vi "Vib Readout.vi"(8 "error in":errorcluster, 11 "DAC HS Vib in":refnum<class "DAC HS Vib.lvclass">) -> (0 "error out":errorcluster, 3 "DAC HS Vib out":refnum<class "DAC HS Vib.lvclass">)   [LabVIEW 2019, in "DAC.lvlib" / "DAC HS Vib.lvclass"]
uses:
  DAC HS Vib.lvclass
  DAC.lvclass
  <vilib>/DAQmx/read.llb/DAQmx Read (Analog DBL 1Chan 1Samp).vi
  <vilib>/DAQmx/read.llb/DAQmx Read (Analog Wfm 1Chan NSamp).vi
  Results/Results Method.ctl
  Results/Results.lvlib
  Results/DeepU Results/DeepU Results.lvclass
  C:/Users/krio/Documents/LV_Projects/test-stand/App/DAC/DAC.lvclass
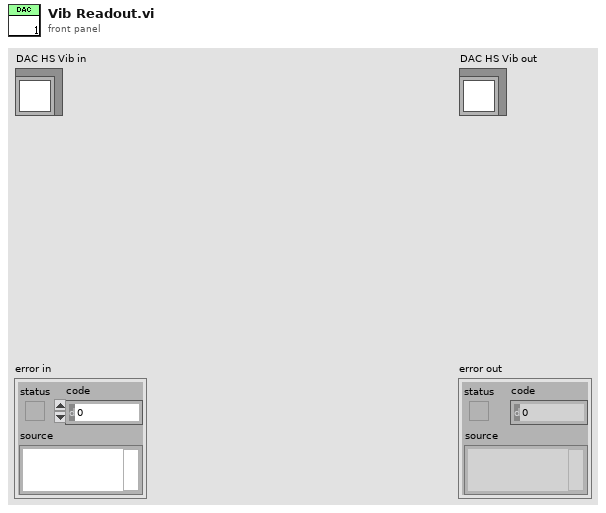
[diagram p1: front panel]
types:
  T1 = typedef "Results.lvlib/Results Method.ctl" = enum16{"Get", "Set"}
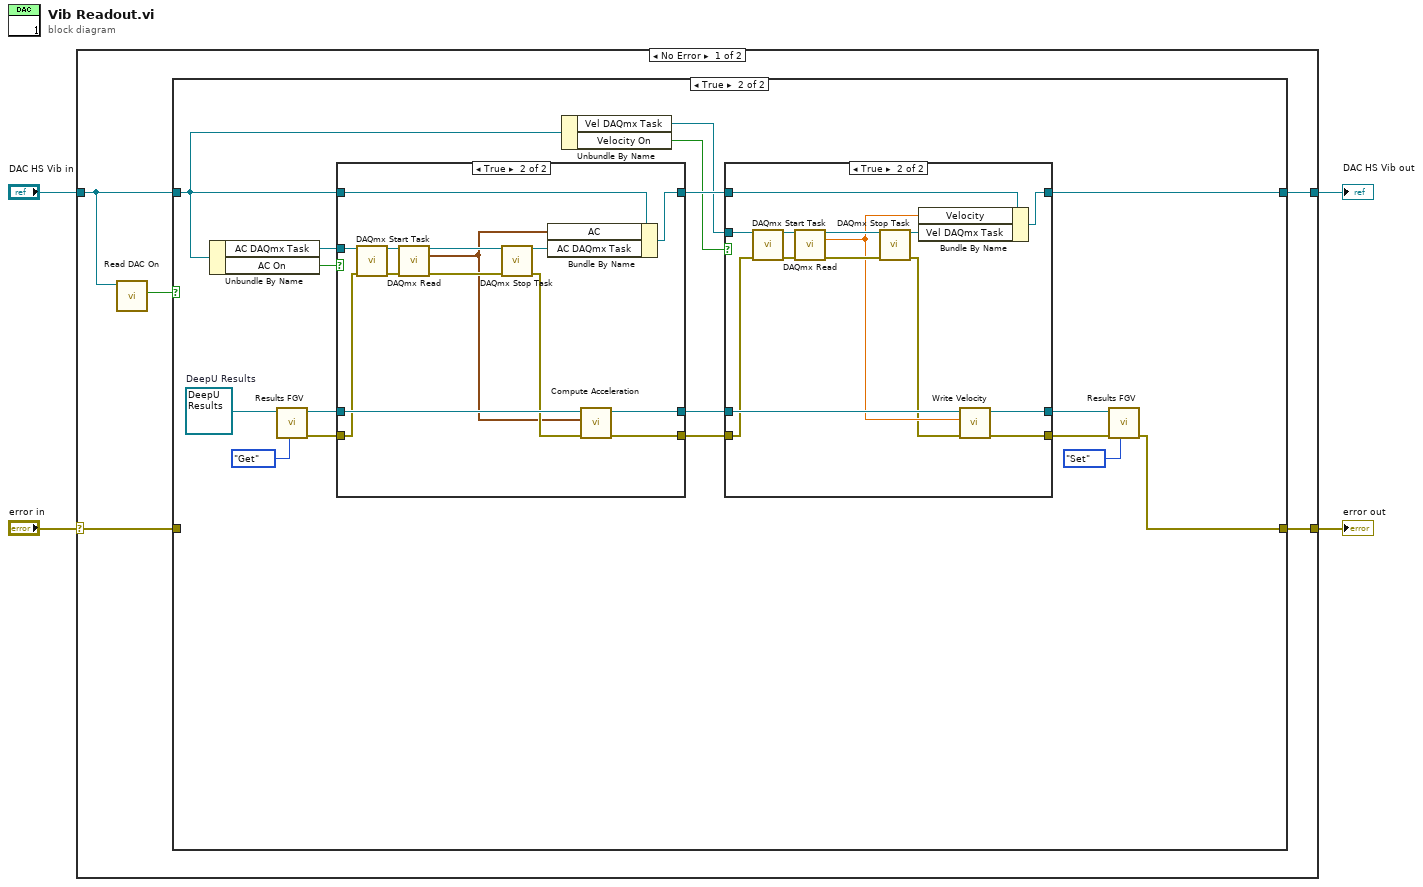
[diagram p0: block diagram]
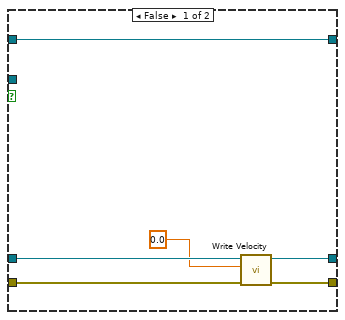
[diagram p3: hidden frame]
diagram:
  n1 = case shown="No Error" "error in" {
    selector: "error in" -> [w5 w67]
    tunnel: [w6 w67] -> w3
    tunnel: [w7 w66] -> w1
    tunnel: "DAC HS Vib in" -> [w8 w66]
    frame No Error {
      n2 = call "Read DAC On.vi"("DAC in"=w8) -> ("DAC On"=w9:bool)  [unwired: 8 in, 2 out]
      n3 = case shown="True" w9 {
        tunnel: w8 -> [w11 w25]
        tunnel: [w11 w27] -> w7
        tunnel: w5 -> [w10 _]
        tunnel: [w10 w15] -> w6
        frame False {
        }
        frame True {
          w21 = refnum<class "DeepU Results.lvclass"> refnum  # DeepU Results
          n4 = Unbundle By Name(w25) -> ("AC DAQmx Task"=w26:refnum<k21>, "AC On"=w24:bool)
          n5 = call-dynamic "Results FGV.vi"("Method"=Results_Method."Get", "DeepU Results in"=w21) -> ("error out"=w12:errorcluster, "DeepU Results out"=w18:refnum<class "DeepU Results.lvclass">)  [unwired: 8 in]
          n6 = case shown="True" w24 {
            tunnel: w25 -> [w51 w65]
            tunnel: [w51 w64] -> w28
            tunnel: w26 -> [_ w63]
            tunnel: w18 -> [w50 w57]
            tunnel: [w50 w56] -> w17
            tunnel: [w49 w54] -> w13
            tunnel: w12 -> [w49 w53]
            frame False {
            }
            frame True {
              n7 = call <vilib>:"DAQmx Start Task.vi"("task/channels in"=w63, "error in"=w53) -> ("task out"=w62:refnum<k21>, "error out"=w59:errorcluster)  [unwired: 12 in]
              n8 = call-poly <vilib>:"DAQmx Read.vi"("task/channels in"=w62, "error in"=w59) -> ("task out"=w61:refnum<k21>, "data"=w52:waveform(dbl), "error out"=w58:errorcluster)  [unwired: 11 in]
              n9 = call <vilib>:"DAQmx Stop Task.vi"("task/channels in"=w61, "error in"=w58) -> ("task out"=w60:refnum<k21>, "error out"=w55:errorcluster)  [unwired: 12 in]
              n10 = Bundle By Name(cluster=w65, "AC"=w52, "AC DAQmx Task"=w60) -> (w64:refnum<class "DAC HS Vib.lvclass">)
              n11 = call "Compute Acceleration.vi"("error in"=w55, "AC"=w52, "DeepU Results in"=w57) -> ("error out"=w54:errorcluster, "DeepU Results out"=w56:refnum<class "DeepU Results.lvclass">)  [unwired: 7 in]
            }
          }
          n12 = Unbundle By Name(w25) -> ("Vel DAQmx Task"=w22:refnum<k21>, "Velocity On"=w23:bool)
          n13 = case shown="True" w23 {
            tunnel: [w34 w48] -> w27
            tunnel: w28 -> [w34 w47]
            tunnel: w22 -> [_ w46]
            tunnel: w17 -> [w33 w40]
            tunnel: [w32 w38] -> w16
            tunnel: [w29 w36] -> w14
            tunnel: w13 -> [w30 w35]
            frame False {
              n14 = call "Write Velocity.vi"("error in (no error)"=w30, "Velocity"=0.0, "DeepU Results in"=w33) -> ("error out"=w29:errorcluster, "DeepU Results out"=w32:refnum<class "DeepU Results.lvclass">)  [unwired: 7 in]
            }
            frame True {
              n15 = call <vilib>:"DAQmx Start Task.vi"("task/channels in"=w46, "error in"=w35) -> ("task out"=w45:refnum<k21>, "error out"=w42:errorcluster)  [unwired: 12 in]
              n16 = call-poly <vilib>:"DAQmx Read.vi"("task/channels in"=w45, "error in"=w42) -> ("task out"=w44:refnum<k21>, "data"=w39:dbl, "error out"=w41:errorcluster)  [unwired: 11 in]
              n17 = call <vilib>:"DAQmx Stop Task.vi"("task/channels in"=w44, "error in"=w41) -> ("task out"=w43:refnum<k21>, "error out"=w37:errorcluster)  [unwired: 12 in]
              n18 = Bundle By Name(cluster=w47, "Velocity"=w39, "Vel DAQmx Task"=w43) -> (w48:refnum<class "DAC HS Vib.lvclass">)
              n19 = call "Write Velocity.vi"("error in (no error)"=w37, "Velocity"=w39, "DeepU Results in"=w40) -> ("error out"=w36:errorcluster, "DeepU Results out"=w38:refnum<class "DeepU Results.lvclass">)  [unwired: 7 in]
            }
          }
          n20 = call-dynamic "Results FGV.vi"("Method"=Results_Method."Set", "error in"=w14, "DeepU Results in"=w16) -> ("error out"=w15:errorcluster)  [unwired: 7 in, 1 out]
        }
      }
    }
    frame Error {
    }
  }
  "error out" <- w3
  "DAC HS Vib out" <- w1
